vi "Do Something Else and Wait for Reply.vi"(8 "error in (no error)":errorcluster, 9 "X":dbl, 10 "Do Something Else Message":string) -> (0 "error out":errorcluster, 1 "timed out?":bool, 2 "Reply Payload":T1)   [LabVIEW 2017, in "My Singleton Module.lvlib"]
doc: "Send the Do Something Else request to the Module's Main.vi.\n_____\nBased on Delacor QMH Project Template 3.1.0.34."
uses:
  My Singleton Module.lvlib
  Do Something Else and Wait (Reply Payload)--cluster.ctl
  Do Something Else and Wait for Reply Argument--cluster.ctl
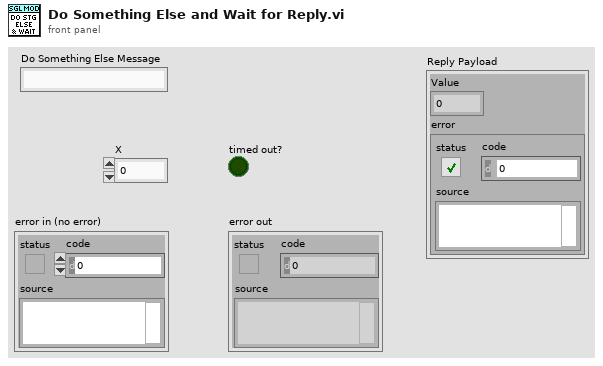
[diagram p1: front panel]
types:
  T1 = typedef "My Singleton Module.lvlib/Do Something Else and Wait (Reply Payload)--cluster.ctl" = cluster{"Value":dbl, "error":errorcluster}
  T2 = typedef "My Singleton Module.lvlib/Request Events--cluster.ctl" = cluster{"Stop Module":refnum<user-event>, "Do Something":refnum<user-event>, "Do Something Else":refnum<user-event>, "Do Something Else and Wait for Reply":refnum<user-event>, "Show Panel":refnum<user-event>, "Hide Panel":refnum<user-event>, "Get Module Execution Status":refnum<user-event>, "Show Diagram":refnum<user-event>}
  T3 = typedef "My Singleton Module.lvlib/Do Something Else and Wait for Reply Argument--cluster.ctl" = cluster{"Do Something Else Msg":string, "X":dbl, "Wait Notifier":refnum<notifier>}
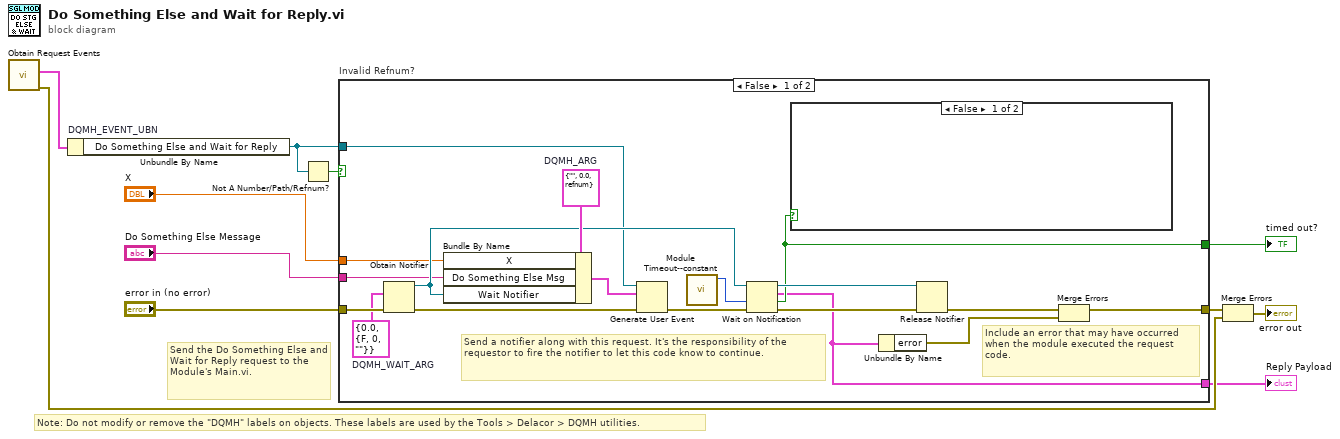
[diagram p0: block diagram]
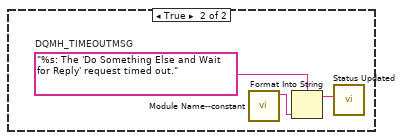
[diagram p2: hidden frame]
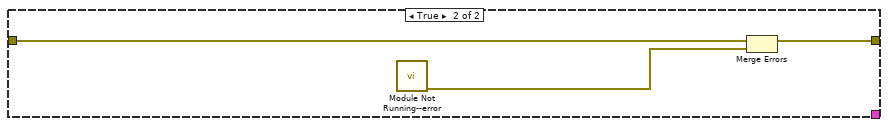
[diagram p3: hidden frame]
diagram:
  # "Note: Do not modify or remove the \"DQMH\" labels on objects. These labels are used by the Tools > Delacor > DQMH utilities."
  # "Send the Do Something Else and Wait for Reply request to the Module's Main.vi."
  n1 = call "Obtain Request Events.vi"() -> ("error out"=w10:errorcluster, "My Singleton Module Request Events"=w9:T2)  [unwired: 10 in]
  n2 = Unbundle By Name "DQMH_EVENT_UBN"(w9) -> ("Do Something Else and Wait for Reply"=w3:refnum<user-event>)
  n3 = Not A Number/Path/Refnum?(number/path/refnum=w3) -> (NaN/Path/Refnum?=w8:bool)
  n4 = case "Invalid Refnum?" shown="False" w8 {
    tunnel: [w14 w34] -> w4
    tunnel: "X" -> [w22 _]
    tunnel: "Do Something Else Message" -> [w21 _]
    tunnel: "error in (no error)" -> [w20 w33]
    tunnel: w3 -> [w19 _]
    tunnel: [w17 _] -> w2
    tunnel: [w13 _] -> w1
    frame False {
      w18 = T1 {"Value"=0.0, "error"={"status"=FALSE, "code"=0, "source"=""}}  # DQMH_WAIT_ARG
      w28 = T3 {"Do Something Else Msg"="", "X"=0.0, "Wait Notifier"=refnum}  # DQMH_ARG
      # "Include an error that may have occurred when the module executed the request code."
      # "Send a notifier along with this request. It's the responsibility of the requestor to fire the notifier to let this code know to continue."
      n5 = Obtain Notifier(notification data type=w18, error in (no error)=w20) -> (notifier out=w25:refnum<notifier>, error out=w26:errorcluster)  [unwired: 2 in, 1 out]
      n6 = Bundle By Name(cluster=w28, "X"=w22, "Do Something Else Msg"=w21, "Wait Notifier"=w25) -> (w27:T3)
      n7 = Generate User Event(user event=w19, event data cluster=w27, error in=w26) -> (error out=w29:errorcluster)  [unwired: 1 in, 1 out]
      n8 = call "Module Timeout--constant.vi"() -> ("Module Timeout"=w24:i32)  [unwired: 11 in]
      n9 = Wait on Notification(notifier=w25, timeout in ms (-1)=w24, error in (no error)=w29) -> (notifier out=w23:refnum<notifier>, notification=w13:T1, timed out?=w17:bool, error out=w16:errorcluster)  [unwired: 1 in]
      n10 = case shown="False" w17 {
        frame False {
        }
        frame True {
          w30 = "%s: The 'Do Something Else and Wait for Reply' request timed out."  # DQMH_TIMEOUTMSG
          n11 = call "Module Name--constant.vi"() -> ("Module Name"=w31:string)  [unwired: 11 in]
          n12 = Format Into String(format string=w30, w31) -> (resulting string=w32:string)  [unwired: 2 in, 1 out]
          n13 = call "Status Updated.vi"("Status"=w32) -> ()  [unwired: 10 in, 1 out]
        }
      }
      n14 = Unbundle By Name(w13) -> ("error"=w12:errorcluster)
      n15 = Release Notifier(notifier=w23, error in (no error)=w16) -> (error out=w15:errorcluster)  [unwired: 1 in, 2 out]
      n16 = Merge Errors(w15, w12) -> (w14:errorcluster)
    }
    frame True {
      n17 = call "Module Not Running--error.vi"() -> ("error out"=w35:errorcluster)  [unwired: 11 in]
      n18 = Merge Errors(w33, w35) -> (w34:errorcluster)
    }
  }
  "timed out?" <- w2
  "Reply Payload" <- w1
  n19 = Merge Errors(w4, w10) -> (→"error out":errorcluster)
